vi "DEMO.vi"() -> ()   [LabVIEW 2024]
uses:
  <instrlib>/EFmeter/EFmeter.lvlib
panel:
  in  "Combo Box":string(combo)="VOLT"
  in  "Ring":u16(ring) items=["CH2"=2, "CH1"=1]
  out "Waveform Graph":dbl[](graph)
  out "error out":errorcluster
  in  "VISA resource name":refnum<visa-resource-name>
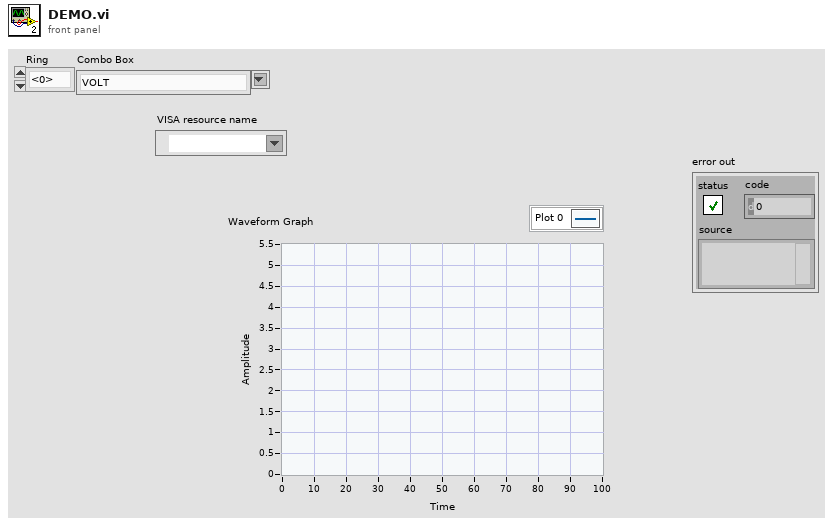
[diagram p1: front panel]
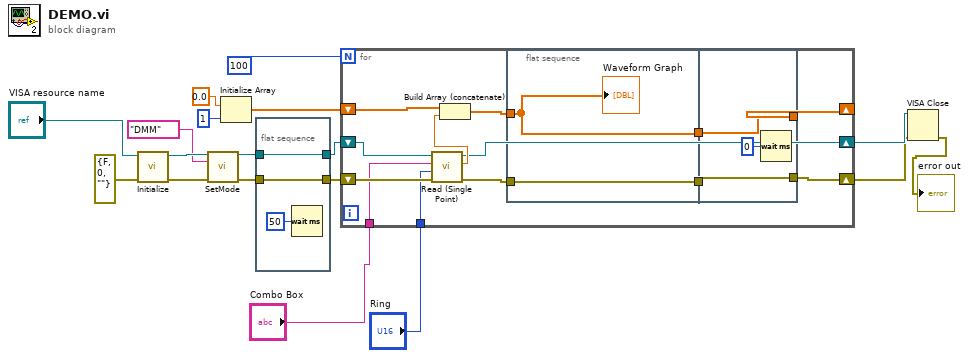
[diagram p0: block diagram]
diagram:
  n1 = call <instrlib>:"Initialize.vi"("error in (no error)"=errorcluster {"status"=FALSE, "code"=0, "source"=""}, "VISA resource name"="VISA resource name") -> ("error out"=w11:errorcluster, "VISA resource name out"=w12:refnum<visa-resource-name>)  [unwired: 8 in]
  n2 = call <instrlib>:"SetMode.vi"("VISA resource name"=w12, "Combo Box"="DMM", "error in (no error)"=w11) -> ("VISA resource name out"=w4:refnum<visa-resource-name>, "error out"=w1:errorcluster)  [unwired: 11 in]
  n3 = Initialize Array(0.0 ("element"), 1 ("dimension size")) -> (w15:dbl[])
  n4 = flat-sequence {
    tunnel: w4 -> [w21]
    tunnel: [w21] -> w3
    tunnel: [w20] -> w2
    tunnel: w1 -> [w20]
    frame #0 {
      n5 = Wait (ms)(milliseconds to wait=u32 50) -> ()  [unwired: 1 out]
    }
  }
  n6 = for {
    N: 100 -> [_]
    shift-right: [w26] -> w6
    shift-left: w2 -> [w34]
    shift-right: [w27] -> _
    shift-left: w15 -> [w32]
    tunnel: "Combo Box" -> [w29]
    tunnel: "Ring" -> [w30]
    shift-right: [w22] -> w7
    shift-left: w3 -> [w33]
    n7 = call <instrlib>:"Read (Single Point).vi"("error in (no error)"=w34, "Ring"=w30, "Combo Box"=w29, "VISA resource name"=w33) -> ("error out"=w25:errorcluster, "Measurement"=w31:dbl, "VISA resource name out"=w22:refnum<visa-resource-name>)  [unwired: 5 in]
    n8 = Build Array (concatenate)(w32, w31) -> (w28:dbl[])
    n9 = flat-sequence {
      tunnel: w25 -> [w36]
      tunnel: w28 -> [w35]
      tunnel: [w35] -> w24
      tunnel: [w36] -> w23
      tunnel: [w39] -> w27
      tunnel: [w38] -> w26
      tunnel: w24 -> [w39]
      tunnel: w23 -> [w38]
      frame #0 {
        "Waveform Graph" <- w35
      }
      frame #1 {
        n10 = Wait (ms)(milliseconds to wait=u32 0) -> ()  [unwired: 1 out]
      }
    }
  }
  n11 = VISA Close(VISA resource name=w7, error in (no error)=w6) -> (error out=→"error out":errorcluster)
